vi "noise_integration.vi"(8 "stop frequency":dbl, 9 "start frequency":dbl, 11 "magnitude":cluster{"f0":dbl, "df":dbl, "magnitude":dbl[]}) -> (2 "rms value":dbl format="%0.2f", 3 "mean":dbl format="%0.2f")   [LabVIEW 2021]
uses:
  <vilib>/Analysis/5stat.llb/RMS (DBL).vi
  <vilib>/Analysis/NI_AALPro.lvlib
panel:
  out "error":i32
  out "Waveform Graph":dbl[](graph)
  out "stop index":dbl
  out "start index":dbl
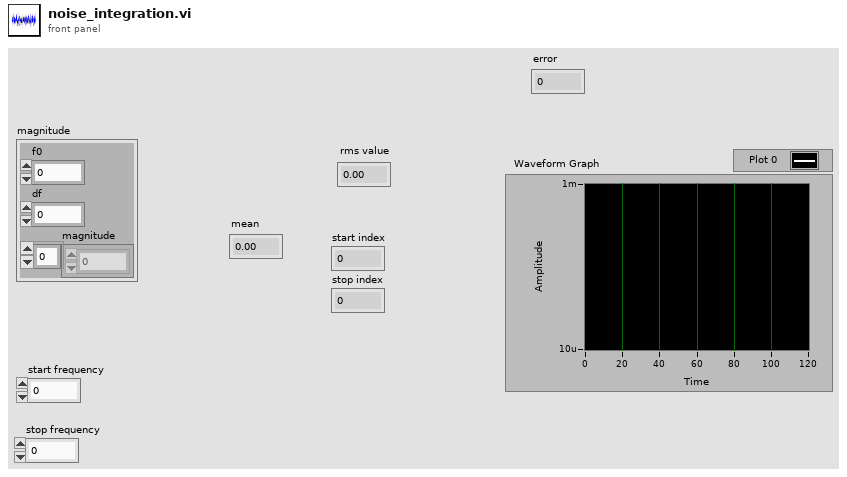
[diagram p1: front panel]
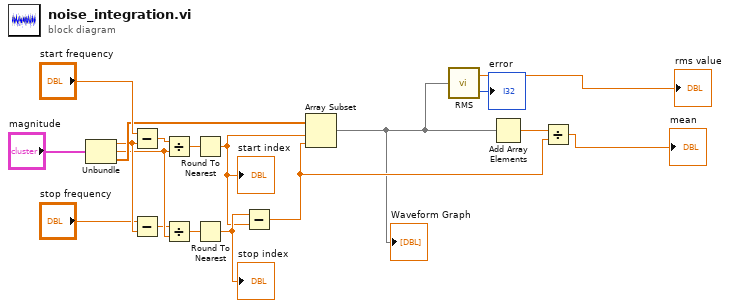
[diagram p0: block diagram]
diagram:
  n1 = Unbundle("magnitude") -> ("f0"=w13:dbl, "df"=w12:dbl, "magnitude"=w14:dbl[])
  n2 = Subtract(x="start frequency", y=w13) -> (x-y=w16:dbl)
  n3 = Subtract(x="stop frequency", y=w13) -> (x-y=w10:dbl)
  n4 = Divide(x=w16, y=w12) -> (x/y=w15:dbl)
  n5 = Divide(x=w10, y=w12) -> (x/y=w9:dbl)
  n6 = Round To Nearest(number=w15) -> (nearest integer value=w7:dbl)
  "start index" <- w7
  n7 = Round To Nearest(number=w9) -> (nearest integer value=w8:dbl)
  "stop index" <- w8
  n8 = Subtract(x=w8, y=w7) -> (x-y=w5:dbl)
  n9 = Array Subset(array=w14, index=w7, length=w5) -> (w3:dbl[])
  "Waveform Graph" <- w3
  n10 = call-poly <vilib>:"RMS.vi"("X"=w3) -> ("rms value"=→"rms value":dbl, "error"=→"error":i32)
  n11 = Add Array Elements(numeric array=w3) -> (sum=w6:dbl)
  n12 = Divide(x=w6, y=w5) -> (x/y=→"mean":dbl)
